vi "Save_to_Project.vi"(8 "error in (no error)":errorcluster, 9 "index":i32, 10 "buildObject":T1, 11 "AB_Source in":refnum<class "AB_Source.lvclass">) -> (0 "error out":errorcluster, 3 "AB_Source out":refnum<class "AB_Source.lvclass">)   [LabVIEW 2020, in "AB_Source.lvclass"]
uses:
  <vilib>/AppBuilder/AB_Classes/Source/AB_Source.lvclass
  <resource>/Framework/Providers/API/ItemRef.ctl
  <vilib>/AppBuilder/AB_Classes/Source/AB_Source.lvclass/AB_Source.ctl
  <vilib>/AppBuilder/RW_Project/AB_RW_Project_Source_Data.ctl
  <vilib>/AppBuilder/AB_Source_Inclusion.ctl
  <vilib>/AppBuilder/AB_Source_Properties.ctl
  <vilib>/AppBuilder/AB_Source_Property_Type.ctl
  <vilib>/AppBuilder/RW_Project/AB_RW_Project_PropBag_Action.ctl
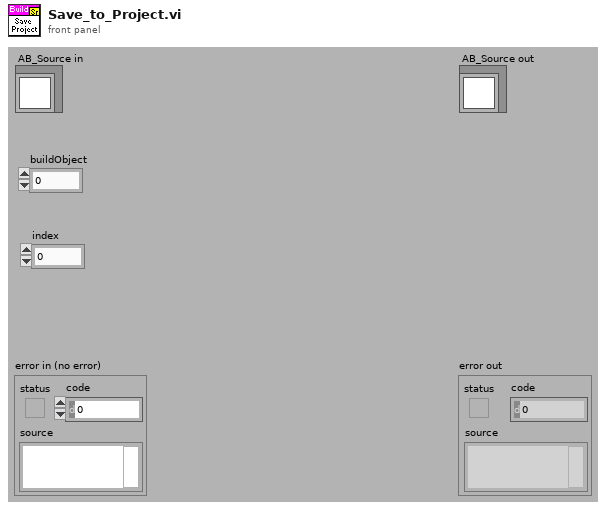
[diagram p1: front panel]
types:
  T1 = typedef "ItemRef.ctl" = u64
  T2 = typedef "AB_RW_Project_Source_Data.ctl" = cluster{"itemID":string, "sourceInclusion":T3, "destinationIndex":i32, "properties":T4[], "newName":string, "lvfile":bool, "preventRename":bool}
  T3 = typedef "AB_Source_Inclusion.ctl" = enum16{"IncludeIfReferenced", "Include", "Exclude", "TopLevel"}
  T4 = typedef "AB_Source_Properties.ctl" = cluster{"sourcePropertyType":T5, "value":variant}
  T5 = typedef "AB_Source_Property_Type.ctl" = enum16{"Remove block diagram", "Remove front panel", "Password", "Window has title bar", "Show menu bar", "Show vertical scroll bar", "Show horizontal scroll bar", "Show toolbar", "Show Abort button", "Show fp when called", "Window behavior", "Allow user to close window", "Window run-time position", "Run when opened", "Allow debugging", "Auto error handling", "Generate guard code", "Use stack variables", "Expression folding", "Integer only", "Inline subVI"}
  T6 = typedef "AB_RW_Project_PropBag_Action.ctl" = enum16{"read", "write", "clear", "readPrevious", "writePrevious", "clearPrevious"}
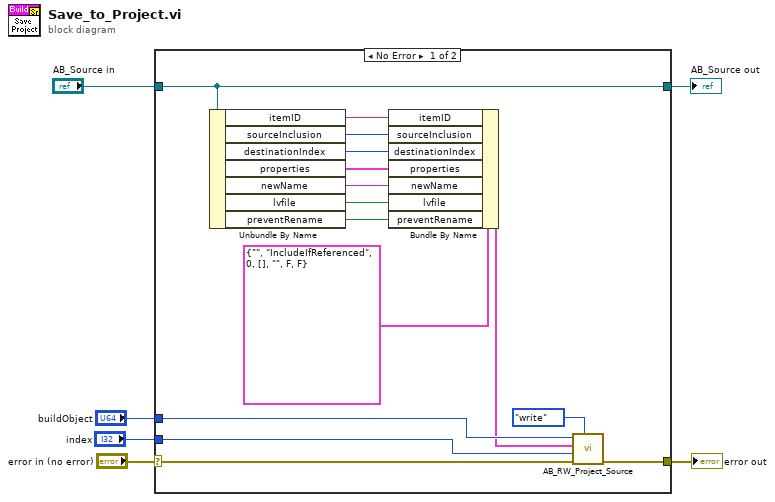
[diagram p0: block diagram]
diagram:
  n1 = case shown="No Error" "error in (no error)" {
    selector: "error in (no error)" -> [w21 w23]
    tunnel: [w20 w23] -> w5
    tunnel: [w17 w22] -> w3
    tunnel: "AB_Source in" -> [w17 w22]
    tunnel: "buildObject" -> [w11 _]
    tunnel: "index" -> [w18 _]
    frame No Error {
      n2 = Unbundle By Name(w17) -> ("itemID"=w15:string, "sourceInclusion"=w14:T3, "destinationIndex"=w13:i32, "properties"=w12:T4[], "newName"=w9:string, "lvfile"=w8:bool, "preventRename"=w7:bool)
      n3 = Bundle By Name(cluster=T2 {"itemID"="", "sourceInclusion"=enum."IncludeIfReferenced", "destinationIndex"=0, "properties"=[], "newName"="", "lvfile"=FALSE, "preventRename"=FALSE} ("dataSource in"), "itemID"=w15, "sourceInclusion"=w14, "destinationIndex"=w13, "properties"=w12, "newName"=w9, "lvfile"=w8, "preventRename"=w7) -> (w10:T2)
      n4 = call <vilib>:"AB_RW_Project_Source.vi"("action"=AB_RW_Project_PropBag_Action."write", "error in (no error)"=w21, "index in"=w18, "dataSource in"=w10, "buildObject"=w11) -> ("error out"=w20:errorcluster)  [unwired: 3 in, 3 out]
    }
    frame Error {
    }
  }
  "error out" <- w5
  "AB_Source out" <- w3
